vi "OldLogReader.vi"() -> ()   [LabVIEW 2011]
doc: "Processes data from status data logs. Requires the user to select the date the log was taken and the log file, then runs through it and finds each time we wrote to the log, and uses the number of times we wrote as the time. It then graphs all the information that is easily graphed and useful. Other data can be obtained by finding it in the case structure in the for loop.\n\n-By Elizabeth Mahon"
uses:
  2-Think/2 Typedefs/Velocity.ctl
  2-Think/2 Typedefs/apparent wind direction.ctl
  2-Think/2 Typedefs/apparent wind speed.ctl
  2-Think/2 Typedefs/apparent wind.ctl
  2-Think/2 Typedefs/heading.ctl
  2-Think/2 Typedefs/UTM Location.ctl
  2-Think/2 Typedefs/robot velocity.ctl
  2-Think/2 Typedefs/rate of turn.ctl
  2-Think/2 Typedefs/pitch and roll.ctl
  2-Think/2 Typedefs/generalized sensor status.ctl
  2-Think/2 Typedefs/indicator LED.ctl
  2-Think/2 Typedefs/Which Boat.ctl
  2-Think/2 Typedefs/absolute wind direction.ctl
  2-Think/2 Typedefs/absolute wind speed.ctl
  0x2-OCU-Think Comm/0x2 Typedefs/Current Waypoint.ctl
  2-Think/2 Typedefs/rudder angle.ctl
  2-Think/2 Typedefs/sail setpt.ctl
  0x2-OCU-Think Comm/0x2 Typedefs/manual override.ctl
  2-Think/2 Typedefs/setpoints to boat.ctl
  0-OCU/0 Typedefs/Maps.ctl
  <vilib>/vision/Image Controls.llb/IMAQ Image.ctl
  0-OCU/0 Typedefs/Apparent Wind Point of Sail.ctl
  0-OCU/0 Typedefs/Sail Position.ctl
  0-OCU/0 Typedefs/Rudder Position.ctl
  2-Think/2 Classes/Waypoint/Waypoint.lvclass
panel:
  in  "Overview Image Ref In":T1
  in  "Stop Replay":bool
  in  "Time":i32(slide) scale=0.0..1698.0
  out "Percent Complete":u8(slide) scale=0.0..100.0
  in  "Stop early":bool
  out "Processing File....":path
  in  "Choose graph to display":T2(tab)
  out "Sense Average":dbl
  out "Code Speed":cluster{i32[], dbl[]}[](graph)
  out "Think Average":dbl
  out "Rudder Manual?":bool
  out "Rudder Position":T3 scale=50.0..-50.0 scale format="%#.2g"
  out "Sail Manual?":bool
  in  "OCU":enum32{"Mission Map", "Detailed Telemetry"}(tab)
  out "Runprotection":bool
  out "Heading":T4 format="%05.1f"
  out "Goodness Functions Polar Plot":picture
  in  "Plot Colors":T5={"Target"=3381759, "No Sail"=16711680, "Change"=16756736, "Pure Waypt"=35080, "Pure Wind"=16860, "Combined"=16777228}
  out "Mission Map":T1(plugin-control)
  out "Apparent Wind Direction\nPoint of Sail":T6 scale=0.0..360.0 scale format="%4d"
  in  "Font Size":i16=40
  in  "Globals":T7(tab)
  out "Don't Tip?":bool
  out "Wind Sensor Status":T8
  out "Robot Heading":T4 format="%05.1f"
  out "Robot UTM Location":T10 {"North" format="%#_10f"; "East" format="%#_8f"}
  out "Robot Velocity":T11
  out "Robot\nRate of Turn":T12 format="%05.1f"
  out "Robot Pitch/Roll":T13 {"Roll" format="%05.1f"; "Pitch" format="%05.1f"}
  out "Robot Speed (m/s)":dbl
  out "Absolute Wind":T14 {"East" format="%#_5g"}
  out "Apparent Wind Direction":T15
  out "Apparent Wind Speed":T16
  out "Apparent Wind":T17
  in  "Map Name":T18="LPB Pool"
  out "Sail Position":T19
  out "Location":cluster{dbl[], dbl[]}[](graph)
  out "Battery Voltage":cluster{i32[], dbl[]}(graph)
  out "Velocity":cluster{i32[], dbl[]}[](graph)
  out "Headings":cluster{i32[], dbl[]}[](graph)
  out "Rudder":cluster{i32[], dbl[]}(graph)
  out "Sail":cluster{i32[], dbl[]}(graph)
  in  "Select date the log was taken":enum32{"Prior to 4/20/2012", "Post 4/20/2012"}(tab)
  in  "Data Log":T28 {"Current Waypoint Coords"."North" format="%#_10f"; "Current Waypoint Coords"."East" format="%#_8f"; "Robot Pitch/Roll"."Roll" format="%05.1f"; "Robot Pitch/Roll"."Pitch" format="%05.1f"; "Robot\nRate of Turn" format="%05.1f"; "Robot\nHeading" format="%05.1f"; "Robot UTM Location"."North" format="%#_10f"; "Robot UTM Location"."East" format="%#_8f"}
  in  "Data Log":T29 {"Current Waypoint Coords"."North" format="%#_10f"; "Current Waypoint Coords"."East" format="%#_8f"; "Robot Pitch/Roll"."Roll" format="%05.1f"; "Robot Pitch/Roll"."Pitch" format="%05.1f"; "Robot\nRate of Turn" format="%05.1f"; "Robot\nHeading" format="%05.1f"; "Robot UTM Location"."North" format="%#_10f"; "Robot UTM Location"."East" format="%#_8f"}
  # "NOTE: This has to be disconnected from the type def, because labview freaks out when the data taken != what this says it should be. Even in little things like type. So depending on how old the data is, you might need to change some things...."
  # "Act and network frequency are always 0.\nAs far as I can tell, network frequency is never set, so of course it's 0.\nAct, while set, is in a sequence structure where the first frame has a while loop that only ends if we e-stop, so it'll never get set."
  # "As Measured"
  # "Where Am I?"
  # "Path Planning"
  # "From Planning Functions"
  # "(this is not a cluster because subitems\nare generated in parallel code)"
  # "NOTE:\n4/20/12 - changed from Timestamp\nto string to record time"
  # "How Am I?"
  # "What's Around Me?"
  # "As Measured"
  # "As Measured"
  # "Loop Rates"
  # "Where Am I?"
  # "Path Planning"
  # "From Planning Functions"
  # "(this is not a cluster because subitems\nare generated in parallel code)"
  # "How Am I?"
  # "What's Around Me?"
  # "As Measured"
  # "As Measured"
  # "Loop Rates"
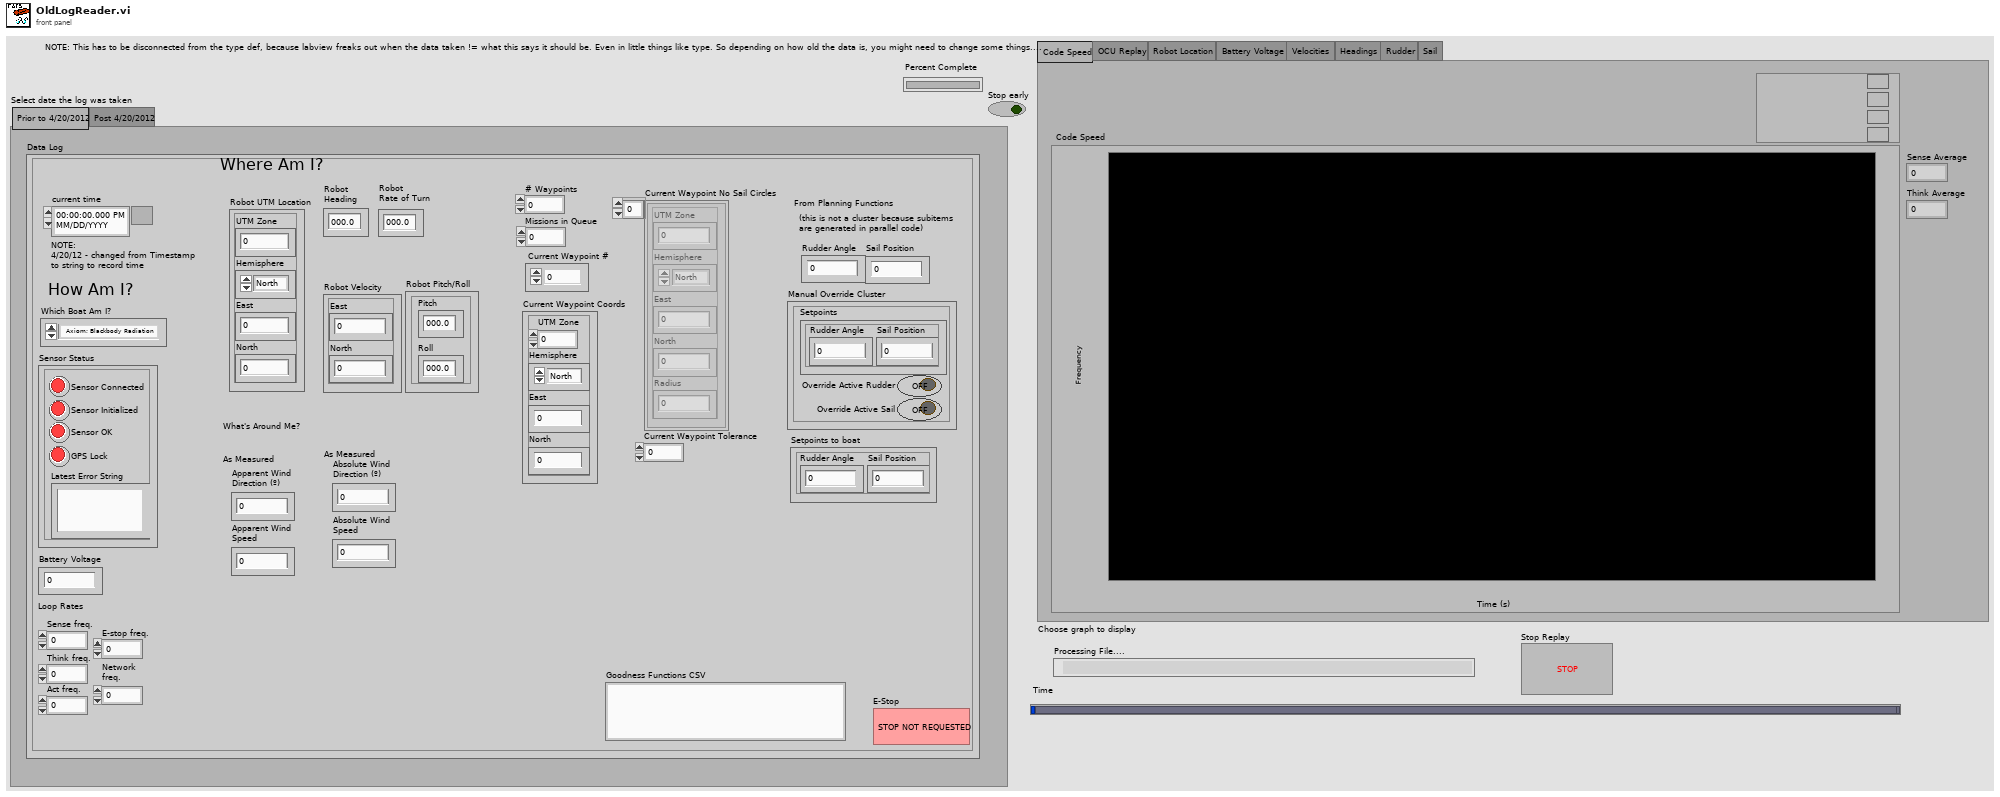
[diagram p1: front panel]
types:
  T1 = typedef "IMAQ Image.ctl" = refnum<image>
  T2 = enum32{"Code Speed", "OCU Replay", "Robot Location", "Battery Voltage", "Velocities", "Headings", "Rudder", "Sail"}
  T3 = typedef "Rudder Position.ctl" = dbl
  T4 = typedef "heading.ctl" = dbl
  T5 = cluster{"Target":u32, "No Sail":u32, "Change":u32, "Pure Waypt":u32, "Pure Wind":u32, "Combined":u32}
  T6 = typedef "Apparent Wind Point of Sail.ctl" = dbl
  T7 = enum32{"How Am I", "Where Am I", "What's Around Me"}
  T8 = typedef "generalized sensor status.ctl" = cluster{"Sensor Connected":T9, "Sensor Initialized":T9, "Sensor OK":T9, "Latest Error String":string, "GPS Lock":T9}
  T9 = typedef "indicator LED.ctl" = bool
  T10 = typedef "UTM Location.ctl" = cluster{"UTM Zone":dbl, "Hemisphere":enum16{"North", "South"}, "East":dbl, "North":dbl}
  T11 = typedef "robot velocity.ctl" = cluster{"East":dbl, "North":dbl}
  T12 = typedef "rate of turn.ctl" = dbl
  T13 = typedef "pitch and roll.ctl" = cluster{"Pitch":dbl, "Roll":dbl}
  T14 = typedef "Velocity.ctl" = cluster{"East":dbl, "North":dbl}
  T15 = typedef "apparent wind direction.ctl" = dbl
  T16 = typedef "apparent wind speed.ctl" = dbl
  T17 = typedef "apparent wind.ctl" = cluster{"Toward Fore":dbl, "Toward Starboard":dbl}
  T18 = typedef "Maps.ctl" = string
  T19 = typedef "Sail Position.ctl" = dbl
  T20 = typedef "Which Boat.ctl" = enum16{"Axiom; Blackbody Radiation", "Simulation"}
  T21 = typedef "absolute wind direction.ctl" = dbl
  T22 = typedef "absolute wind speed.ctl" = dbl
  T23 = typedef "Current Waypoint.ctl" = i32
  T24 = typedef "rudder angle.ctl" = dbl
  T25 = typedef "sail setpt.ctl" = dbl
  T26 = typedef "manual override.ctl" = cluster{"Override Active Rudder":bool, "Setpoints":T27, "Override Active Sail":bool}
  T27 = typedef "setpoints to boat.ctl" = cluster{"Sail Position":T25, "Rudder Angle":T24}
  T28 = cluster{"current time":timestamp, "Which Boat Am I?":T20, "Robot UTM Location":cluster{"UTM Zone":dbl, "Hemisphere":enum16{"North", "South"}, "East":dbl, "North":dbl}, "Robot\nHeading ":T4, "Robot\nRate of Turn":T12, "Robot Velocity":cluster{"East":dbl, "North":dbl}, "Robot Pitch/Roll":cluster{"Pitch":dbl, "Roll":dbl}, "Sensor Status":T8, "Battery Voltage":dbl, "Sense freq.":dbl, "Think freq.":dbl, "Act freq.":dbl, "E-stop freq.":dbl, "Network \nfreq.":dbl, "Apparent Wind\nDirection (º)":T15, "Apparent Wind\nSpeed":T16, "Absolute Wind\nDirection (º)":T21, "Absolute Wind\nSpeed":T22, "Missions in Queue":i32, "# Waypoints":i32, " Current Waypoint #":T23, "Current Waypoint Coords":cluster{"UTM Zone":dbl, "Hemisphere":enum16{"North", "South"}, "East":dbl, "North":dbl}, "Current Waypoint Tolerance":dbl, "Current Waypoint No Sail Circles":cluster{"UTM Zone":dbl, "Hemisphere":enum16{"North", "South"}, "East":dbl, "North":dbl, "Radius":dbl}[], "Rudder Angle":T24, "Sail Position":T25, "Manual Override Cluster":T26, "Setpoints to boat":T27, "E-Stop":bool, "Goodness Functions CSV":string}
  T29 = cluster{"Which Boat Am I?":enum16{"Competition Boat", "Small RC", "Simulation"}, "Robot UTM Location":cluster{"UTM Zone":dbl, "Hemisphere":enum16{"North", "South"}, "East":dbl, "North":dbl}, "Robot\nHeading ":T4, "Robot\nRate of Turn":T12, "Robot Velocity":cluster{"East":dbl, "North":dbl}, "Robot Pitch/Roll":cluster{"Pitch":dbl, "Roll":dbl}, "Sensor Status":T8, "Battery Voltage":dbl, "Sense freq.":dbl, "Think freq.":dbl, "Act freq.":dbl, "E-stop freq.":dbl, "Network \nfreq.":dbl, "Apparent Wind\nDirection (º)":T15, "Apparent Wind\nSpeed":T16, "Absolute Wind\nDirection (º)":T21, "Absolute Wind\nSpeed":T22, "Missions in Queue":i32, "# Waypoints":i32, " Current Waypoint #":T23, "Current Waypoint Coords":cluster{"UTM Zone":dbl, "Hemisphere":enum16{"North", "South"}, "East":dbl, "North":dbl}, "Current Waypoint Tolerance":dbl, "Current Waypoint No Sail Circles":cluster{"UTM Zone":dbl, "Hemisphere":enum16{"North", "South"}, "East":dbl, "North":dbl, "Radius":dbl}[], "Rudder Angle":T24, "Sail Position":T25, "Manual Override Cluster":T26, "Setpoints to boat":T27, "E-Stop":bool, "Goodness Functions CSV":string, "Date":string, "Time":string, "Run Protect":bool}
  T30 = cluster{"UTM Zone":dbl, "Hemisphere":enum16{"North", "South"}, "East":dbl, "North":dbl}
  T31 = cluster{"UTM Zone":dbl, "Hemisphere":enum16{"North", "South"}, "East":dbl, "North":dbl, "Radius":dbl}[]
  T32 = cluster{"UTM Zone":bool, "Hemisphere":bool, "East":bool, "North":bool}
  T33 = typedef "0-Image Descriptor.ctl" = cluster{"Upper-Left Corner Coordinates":T10, "Meters/Pixel":dbl}
  T34 = cluster{"Image Ref Out":T1, "Image Descriptor":T33}
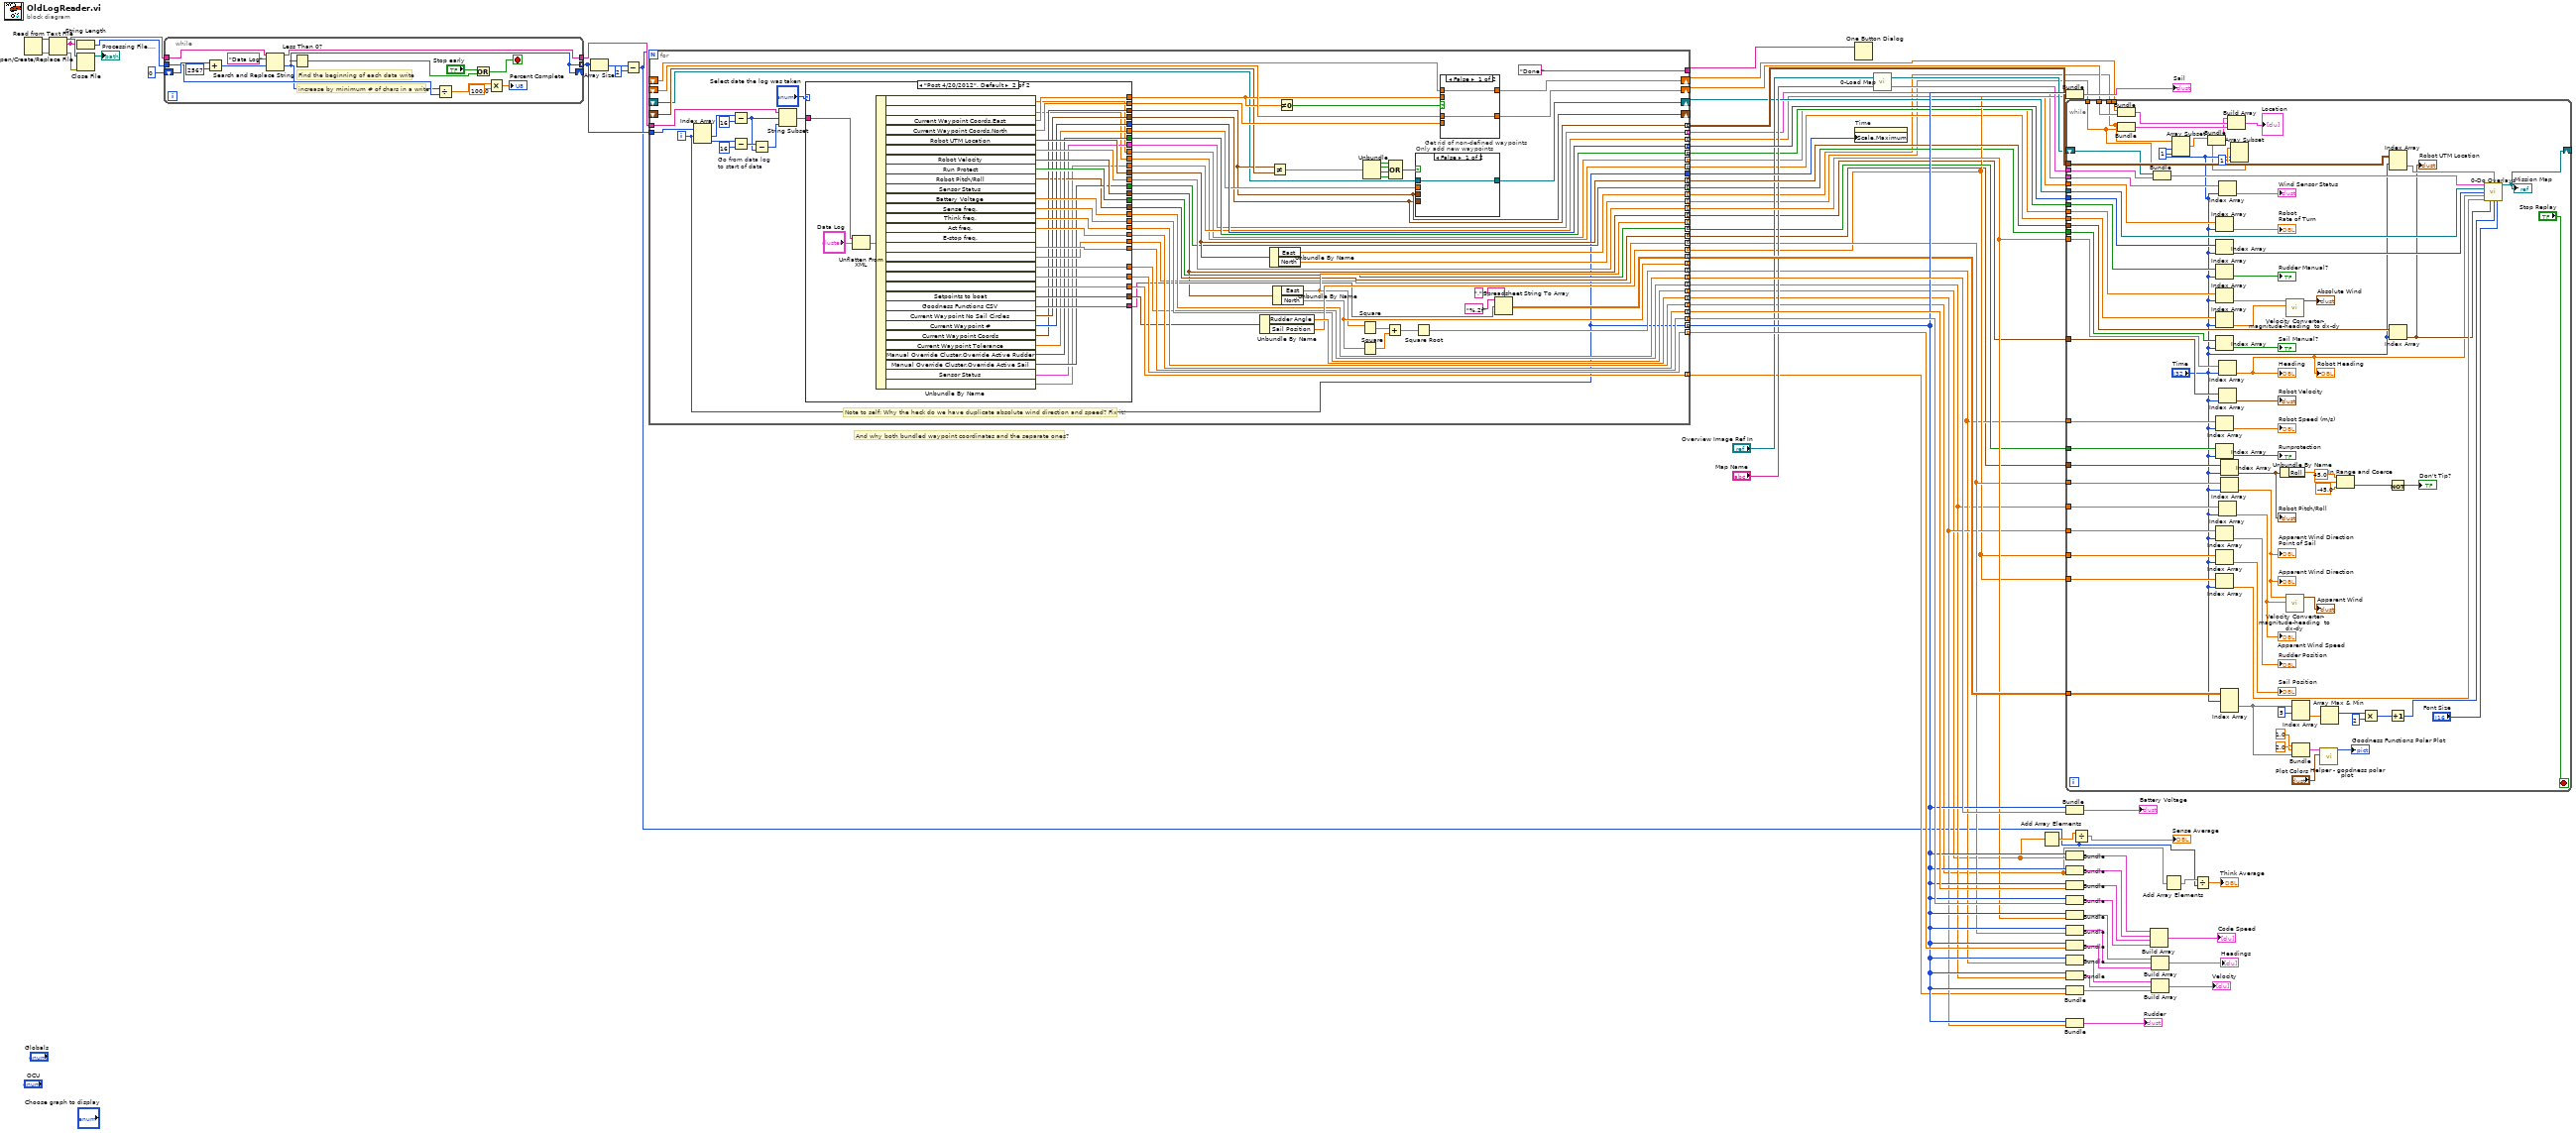
[diagram p0: block diagram]
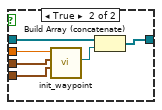
[diagram p2: hidden frame]
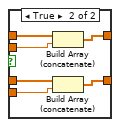
[diagram p3: hidden frame]
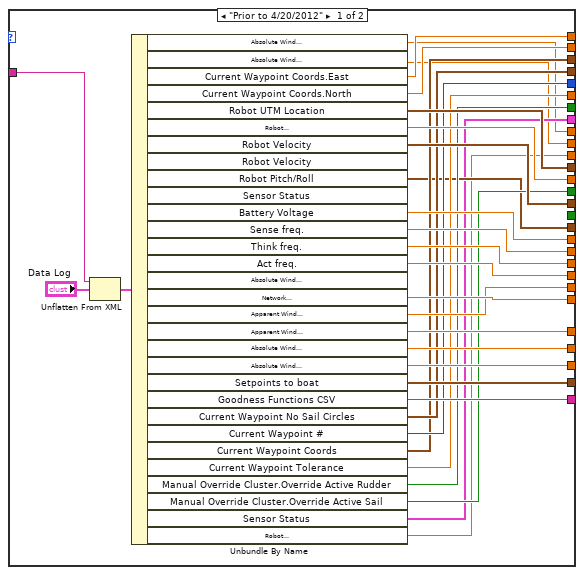
[diagram p4: hidden frame]
diagram:
  # "And why both bundled waypoint coordinates and the separate ones?"
  n1 = Open/Create/Replace File() -> (refnum out=w71:refnum<file>, error out=w42:errorcluster)  [unwired: 6 in, 1 out]
  n2 = Read from Text File(file (use dialog)=w71, error in=w42) -> (refnum out=w43:refnum<file>, text=w37:string, error out=w44:errorcluster)  [unwired: 2 in, 1 out]
  n3 = String Length(string=w37) -> (length=w36:i32)
  n4 = Close File(refnum=w43, error in=w44) -> (path=→"Processing File....":path)  [unwired: 1 out]
  n5 = while {
    tunnel: w37 -> [w75]
    shift-right: [w73] -> _
    shift-left: 0 ("offset past replacement") -> [w85]
    tunnel: [w74] -> w69
    tunnel: [w73] -> w40 mode=indexing
    tunnel: w36 -> [w77]
    stop <- w83 stop-if-true
    # "increase by minimum # of chars in a write"
    # "Find the beginning of each data write"
    n6 = Add(x=w85, y=2567) -> (x+y=w76:i32)
    n7 = Search and Replace String(input string=w75, search string="Data Log", offset=w76) -> (result string=w74:string, offset past replacement=w73:i32)  [unwired: 5 in, 2 out]
    n8 = Less Than 0?(x=w73) -> (x < 0?=w81:bool)
    n9 = Divide(x=w73, y=w77) -> (x/y=w80:dbl)
    n10 = Or(x="Stop early", y=w81) -> (x .or. y?=w83:bool)
    n11 = Multiply(x=w80, y=100.0) -> (x*y=→"Percent Complete":dbl)
  }
  n12 = Array Size(array=w40) -> (size(s)=w68:i32)
  n13 = Subtract(x=w68, y=2) -> (x-y=w2:i32)
  n14 = for {
    N: w2 -> [_]
    tunnel: w40 -> [w145]
    tunnel: w69 -> [w148]
    tunnel: [w131] -> w33 mode=indexing
    tunnel: [w130] -> w56 mode=indexing
    tunnel: [w129] -> w7 mode=indexing
    tunnel: [w128] -> w4 mode=indexing
    tunnel: [w127] -> w54 mode=indexing
    tunnel: [w126] -> w53 mode=indexing
    tunnel: [w123] -> w27 mode=indexing
    tunnel: [w125] -> w19 mode=indexing
    tunnel: [w122] -> w50 mode=indexing
    tunnel: [w124] -> w18 mode=indexing
    tunnel: [w86] -> w45 mode=indexing
    tunnel: [w141] -> w20 mode=indexing
    tunnel: [w140] -> w24 mode=indexing
    tunnel: [w139] -> w23 mode=indexing
    tunnel: [w138] -> w9 mode=indexing
    tunnel: [w137] -> w8 mode=indexing
    tunnel: ["Done!"] -> w46
    tunnel: [w135] -> _ mode=indexing
    tunnel: [w134] -> _ mode=indexing
    tunnel: [w120] -> w26 mode=indexing
    tunnel: [w116] -> w39 mode=indexing
    tunnel: [w86] -> w38
    shift-right: [w113] -> w10
    shift-left: _ -> [w112]
    shift-right: [w110] -> w11
    shift-left: _ -> [w109]
    tunnel: [w97] -> w35 mode=indexing
    tunnel: [w108] -> w34 mode=indexing
    tunnel: [w107] -> w32 mode=indexing
    shift-right: [w98] -> _
    shift-left: _ -> [w106]
    shift-right: [w96] -> w25
    shift-left: _ -> [w95]
    tunnel: [w94] -> w22 mode=indexing
    tunnel: [w93] -> w21 mode=indexing
    tunnel: [w92] -> w17 mode=indexing
    tunnel: [w91] -> w16 mode=indexing
    tunnel: [w90] -> w15 mode=indexing
    tunnel: [w89] -> w14 mode=indexing
    tunnel: [w88] -> w13 mode=indexing
    tunnel: [w87] -> w12 mode=indexing
    i -> [w86]
    # "Note to self: Why the heck do we have duplicate absolute wind direction and speed? Fix it!"
    n15 = Index Array(array=w145, index #1=w86) -> (element #1=w153:i32, element #2=w151:i32)  [unwired: 1 in]
    n16 = Subtract(x=w153, y=16) -> (x-y=w146:i32)
    n17 = Subtract "Go from data log\nto start of data"(x=w151, y=16) -> (x-y=w149:i32)
    n18 = Subtract(x=w149, y=w146) -> (x-y=w147:i32)
    n19 = String Subset(string=w148, offset (0)=w146, length (rest)=w147) -> (substring=w132:string)
    n20 = case shown="\"Post 4/20/2012\", Default" "Select date the log was taken" {
      tunnel: w132 -> [w197 w227]
      tunnel: [w196 w226] -> w107
      tunnel: [w195 w225] -> w131
      tunnel: [w194 w224] -> w90
      tunnel: [w193 w223] -> w130
      tunnel: [w192 w222] -> w129
      tunnel: [w191 w221] -> w128
      tunnel: [w190 w220] -> w127
      tunnel: [w189 w219] -> w126
      tunnel: [w188 w217] -> w125
      tunnel: [w187 w215] -> w124
      tunnel: [w186 w218] -> w123
      tunnel: [w185 w216] -> w122
      tunnel: [w183 w214] -> w121
      tunnel: [_ w213] -> w120
      tunnel: [w182 w212] -> w119
      tunnel: [w181 w211] -> w111
      tunnel: [w180 w210] -> w114
      tunnel: [w179 w209] -> w97
      tunnel: [w178 w208] -> w108
      tunnel: [w177 w207] -> w98
      tunnel: [w176 w206] -> w99
      tunnel: [w175 w205] -> w94
      tunnel: [w174 w204] -> w93
      tunnel: [w173 w203] -> w92
      tunnel: [w172 w202] -> w91
      tunnel: [w171 w201] -> w89
      tunnel: [w170 w200] -> w88
      tunnel: [w169 w199] -> w87
      frame "Prior to 4/20/2012" {
        n21 = Unflatten From XML(xml string=w197, type="Data Log") -> (value=w184:T28)  [unwired: 1 in, 1 out]
        n22 = Unbundle By Name(w184) -> ("Absolute Wind\nDirection (º)"=w170:T21, "Absolute Wind\nSpeed"=w169:T22, "Current Waypoint Coords.East"=w181:dbl, "Current Waypoint Coords.North"=w180:dbl, "Robot UTM Location"=w196:T30, "Robot\nHeading"=w195:T4, "Robot Velocity"=w194:cluster{"East":dbl, "North":dbl}, "Robot Pitch/Roll"=w173:cluster{"Pitch":dbl, "Roll":dbl}, "Battery Voltage"=w193:dbl, "Sense freq."=w192:dbl, "Think freq."=w191:dbl, "Act freq."=w190:dbl, "Network \nfreq."=w189:dbl, "Apparent Wind\nDirection (º)"=w186:T15, "Apparent Wind\nSpeed"=w188:T16, "Absolute Wind\nDirection (º)"=w185:T21, "Absolute Wind\nSpeed"=w187:T22, "Setpoints to boat"=w183:T27, "Goodness Functions CSV"=w182:string, "Current Waypoint No Sail Circles"=w179:T31, "Current Waypoint #"=w178:T23, "Current Waypoint Coords"=w177:T30, "Current Waypoint Tolerance"=w176:dbl, "Manual Override Cluster.Override Active Rudder"=w175:bool, "Manual Override Cluster.Override Active Sail"=w174:bool, "Sensor Status"=w172:T8, "Robot\nRate of Turn"=w171:T12)  [unwired: 3 out]
      }
      frame "Post 4/20/2012", Default {
        n23 = Unflatten From XML(xml string=w227, type="Data Log") -> (value=w229:T29)  [unwired: 1 in, 1 out]
        n24 = Unbundle By Name(w229) -> ("Absolute Wind\nDirection (º)"=w200:T21, "Absolute Wind\nSpeed"=w199:T22, "Current Waypoint Coords.East"=w211:dbl, "Current Waypoint Coords.North"=w210:dbl, "Robot UTM Location"=w226:T30, "Robot\nHeading"=w225:T4, "Robot Velocity"=w224:cluster{"East":dbl, "North":dbl}, "Run Protect"=w213:bool, "Robot Pitch/Roll"=w203:cluster{"Pitch":dbl, "Roll":dbl}, "Battery Voltage"=w223:dbl, "Sense freq."=w222:dbl, "Think freq."=w221:dbl, "Act freq."=w220:dbl, "Network \nfreq."=w219:dbl, "Apparent Wind\nDirection (º)"=w218:T15, "Apparent Wind\nSpeed"=w217:T16, "Absolute Wind\nDirection (º)"=w216:T21, "Absolute Wind\nSpeed"=w215:T22, "Setpoints to boat"=w214:T27, "Goodness Functions CSV"=w212:string, "Current Waypoint No Sail Circles"=w209:T31, "Current Waypoint #"=w208:T23, "Current Waypoint Coords"=w207:T30, "Current Waypoint Tolerance"=w206:dbl, "Manual Override Cluster.Override Active Rudder"=w205:bool, "Manual Override Cluster.Override Active Sail"=w204:bool, "Sensor Status"=w202:T8, "Robot\nRate of Turn"=w201:T12)  [unwired: 2 out]
      }
    }
    n25 = Unbundle By Name(w121) -> ("Rudder Angle"=w140:T24, "Sail Position"=w139:T25)
    n26 = Unbundle By Name(w107) -> ("East"=w138:dbl, "North"=w137:dbl)
    n27 = Not Equal?(x=w98, y=w106) -> (x != y?=w105:T32)
    n28 = Unbundle By Name(w90) -> ("East"=w134:dbl, "North"=w135:dbl)
    n29 = Not Equal To 0?(x=w111) -> (x != 0?=w115:bool)
    n30 = Square(x=w134) -> (x^2=w143:dbl)
    n31 = Square(x=w135) -> (x^2=w142:dbl)
    n32 = Unbundle(w105) -> ("UTM Zone"=w104:bool, "Hemisphere"=w103:bool, "East"=w102:bool, "North"=w101:bool)
    n33 = Add(x=w143, y=w142) -> (x+y=w144:dbl)
    n34 = Compound Arithmetic op=OR(w104, w103, w102, w101) -> (w100:bool)
    n35 = Square Root(x=w144) -> (sqrt(x)=w141:dbl)
    n36 = case "Only add new waypoints" shown="False" w100 {
      tunnel: w99 -> [_ w160]
      tunnel: w98 -> [_ w159]
      tunnel: w97 -> [_ w158]
      tunnel: [w154 w156] -> w96
      tunnel: w95 -> [w154 w155]
      frame False {
      }
      frame True {
        n37 = call "init_waypoint.vi"("No Sail Circles"=w158, "Coords"=w159, "Tolerance (m)"=w160) -> ("Waypoint Out"=w157:refnum<class "Waypoint.lvclass">)  [unwired: 8 in]
        n38 = Build Array (concatenate)(w155, w157) -> (w156:refnum<class "Waypoint.lvclass">[])
      }
    }
    n39 = case "Get rid of non-defined waypoints" shown="False" w115 {
      tunnel: w114 -> [_ w168]
      tunnel: [w161 w167] -> w113
      tunnel: w112 -> [w161 w166]
      tunnel: w111 -> [_ w165]
      tunnel: [w162 w164] -> w110
      tunnel: w109 -> [w162 w163]
      frame False {
      }
      frame True {
        n40 = Build Array (concatenate)(w163, w165) -> (w164:dbl[])
        n41 = Build Array (concatenate)(w166, w168) -> (w167:dbl[])
      }
    }
    n42 = Spreadsheet String To Array(delimiter (Tab)=",", format string="%.2f", spreadsheet string=w119) -> (array=w116:dbl[][])  [unwired: 1 in]
  }
  n43 = One Button Dialog(message=w46) -> ()  [unwired: 1 in, 1 out]
  n44 = property on="Time" class="Slide (strict)"("Scale.Maximum"=w38) -> ()  [unwired: 2 in, 2 out]
  n45 = call "0-Load Map.vi"("Map Name"="Map Name", "Image Ref In"="Overview Image Ref In") -> ("Image Descriptor"=w30:T33, "Image Ref Out"=w28:T1)
  n46 = Add Array Elements(numeric array=w7) -> (sum=w6:dbl)
  n47 = Bundle(w45, w23) -> (→"Sail":cluster{i32[], T25[]})  [unwired: 1 in]
  n48 = while {
    tunnel: w39 -> [w307]
    tunnel: w35 -> [w300]
    tunnel: w34 -> [w297]
    tunnel: w33 -> [w295]
    tunnel: w23 -> [w294]
    tunnel: w32 -> [w292]
    shift-right: [w284] -> _
    shift-left: w28 -> [w282]
    tunnel: w30 -> [w283]
    tunnel: w27 -> [w281]
    tunnel: w26 -> [w280]
    tunnel: w25 -> [w278]
    tunnel: w24 -> [w276]
    tunnel: w23 -> [w274]
    tunnel: w22 -> [w272]
    tunnel: w21 -> [w270]
    tunnel: w20 -> [w266]
    tunnel: w19 -> [w264]
    tunnel: w17 -> [w263]
    tunnel: w16 -> [w256]
    tunnel: w15 -> [w254]
    tunnel: w14 -> [w252]
    tunnel: w13 -> [w247]
    tunnel: w12 -> [w246]
    tunnel: w11 -> [w239]
    tunnel: w10 -> [w238]
    tunnel: w9 -> [w237]
    tunnel: w8 -> [w234]
    stop <- "Stop Replay" stop-if-true
    n49 = Bundle(w239, w238) -> (w241:cluster{dbl[], dbl[]})  [unwired: 1 in]
    n50 = Bundle(w237, w234) -> (w242:cluster{dbl[], dbl[]})  [unwired: 1 in]
    n51 = Bundle("Image Ref Out"=w282, "Image Descriptor"=w283) -> (w298:T34)  [unwired: 1 in]
    n52 = Array Subset(array=w237, index="Time", length=1) -> (w235:dbl[])
    n53 = Index Array(array=w252, index="Time") -> (element=→"Robot\nRate of Turn":T12)
    n54 = Index Array(array=w297, index="Time") -> (element=w296:T23)
    n55 = Index Array(array=w272, index="Time") -> (element=→"Rudder Manual?":bool)
    n56 = Index Array(array=w247, index="Time") -> (element=w245:T21)
    n57 = Index Array(array=w246, index="Time") -> (element=w244:T22)
    n58 = Index Array(array=w270, index="Time") -> (element=→"Sail Manual?":bool)
    n59 = Index Array(array=w266, index="Time") -> (element=→"Robot Speed (m/s)":dbl)
    n60 = Index Array(array=w280, index="Time") -> (element=→"Runprotection":bool)
    n61 = Index Array(array=w276, index="Time") -> (element=→"Rudder Position":T24)
    n62 = Index Array(array=w274, index="Time") -> (element=→"Sail Position":T25)
    n63 = Index Array(array=w294, index="Time") -> (element=w293:T25)
    n64 = Index Array(array=w256, index="Time") -> (element=→"Wind Sensor Status":T8)
    n65 = Index Array(array=w254, index="Time") -> (element=→"Robot Velocity":cluster{"East":dbl, "North":dbl})
    n66 = Index Array(array=w295, index="Time") -> (element=w267:T4)
    "Heading" <- w267
    "Robot Heading" <- w267
    n67 = Index Array(array=w264, index="Time") -> (element=w248:T16)
    "Apparent Wind Speed" <- w248
    n68 = Index Array(array=w281, index="Time") -> (element=w249:T15)
    "Apparent Wind Direction\nPoint of Sail" <- w249
    "Apparent Wind Direction" <- w249
    n69 = Index Array(array=w263, index="Time") -> (element=w262:cluster{"Pitch":dbl, "Roll":dbl})
    "Robot Pitch/Roll" <- w262
    n70 = Index Array(array=w307, index (dim 0)="Time") -> (element=w291:dbl[][])  [unwired: 2 in]
    n71 = Array Subset(array=w234, index="Time", length=1) -> (w231:dbl[])
    n72 = Bundle(w235, w231) -> (w230:cluster{dbl[], dbl[]})  [unwired: 1 in]
    n73 = Build Array(w230, w241, w242) -> (→"Location":cluster{dbl[], dbl[]}[])
    n74 = Unbundle By Name(w262) -> ("Roll"=w261:dbl)
    n75 = call "Velocity Converter- magnitude-heading  to dx-dy.vi"("Magnitude"=w244, "Heading"=w245) -> ("Vector Out"=→"Absolute Wind":T14)  [unwired: 9 in]
    n76 = call "Velocity Converter- magnitude-heading  to dx-dy.vi"("Magnitude"=w248, "Heading"=w249) -> ("Vector Out"=→"Apparent Wind":T14)  [unwired: 9 in]
    n77 = Index Array(array=w291, index (row)=5 ("disabled index (col)")) -> (element=w290:dbl[])  [unwired: 1 in]
    n78 = Bundle(1.0, 2.0, w291) -> (w303:cluster{dbl, dbl, dbl[][]})  [unwired: 1 in]
    n79 = call "Helper - goodness polar plot.vi"("Plot Colors"="Plot Colors", "Goodness Fns In"=w303) -> ("Goodness Functions Polar Plot"=→"Goodness Functions Polar Plot":picture)  [unwired: 9 in]
    n80 = Array Max & Min(array=w290) -> (max index (indices)=w289:i32)  [unwired: 3 out]
    n81 = In Range and Coerce(upper limit=45.0, x=w261, lower limit=-45.0) -> (In Range?=w258:bool)  [unwired: 1 out]
    n82 = Multiply(x=w289, y=2) -> (x*y=w287:i32)
    n83 = Not(x=w258) -> (.not. x?=→"Don't Tip?":bool)
    n84 = Increment(x=w287) -> (x+1=w286:i32)
    n85 = Index Array(array=w300, index (row)="Time") -> (element=w299:T31)  [unwired: 1 in]
    n86 = Index Array(array=w292, index="Time") -> (element=w268:T30)
    "Robot UTM Location" <- w268
    n87 = call "0-Do Overlays.vi"("Image Reference\nand Descriptor"=w298, "No Sail Circles"=w299, "Waypoints"=w278, "Current Waypoint #"=w296, "Heading"=w267, "Sail Position"=w293, "Robot UTM Location"=w268, "Optimal Heading"=w286, "Font Size"="Font Size") -> ("Image out"=w284:T1)  [unwired: 6 in]
    "Mission Map" <- w284
  }
  n88 = Bundle(w45, w56) -> (→"Battery Voltage":cluster{i32[], dbl[]})  [unwired: 1 in]
  n89 = Bundle(w45, w7) -> (w58:cluster{i32[], dbl[]})  [unwired: 1 in]
  n90 = Bundle(w45, w4) -> (w57:cluster{i32[], dbl[]})  [unwired: 1 in]
  n91 = Bundle(w45, w54) -> (w60:cluster{i32[], dbl[]})  [unwired: 1 in]
  n92 = Bundle(w45, w53) -> (w59:cluster{i32[], dbl[]})  [unwired: 1 in]
  n93 = Bundle(w45, w33) -> (w61:cluster{i32[], T4[]})  [unwired: 1 in]
  n94 = Bundle(w45, w27) -> (w62:cluster{i32[], T15[]})  [unwired: 1 in]
  n95 = Bundle(w45, w50) -> (w63:cluster{i32[], T21[]})  [unwired: 1 in]
  n96 = Bundle(w45, w20) -> (w64:cluster{i32[], dbl[]})  [unwired: 1 in]
  n97 = Bundle(w45, w19) -> (w65:cluster{i32[], T16[]})  [unwired: 1 in]
  n98 = Bundle(w45, w18) -> (w66:cluster{i32[], T22[]})  [unwired: 1 in]
  n99 = Bundle(w45, w24) -> (→"Rudder":cluster{i32[], T24[]})  [unwired: 1 in]
  n100 = Divide(x=w6, y=w2) -> (x/y=→"Sense Average":dbl)
  n101 = Build Array(w58, w57, w60, w59) -> (→"Code Speed":cluster{i32[], dbl[]}[])
  n102 = Build Array(w61, w62, w63) -> (→"Headings":cluster{i32[], T21[]}[])
  n103 = Build Array(w64, w65, w66) -> (→"Velocity":cluster{i32[], T22[]}[])
  n104 = Add Array Elements(numeric array=w4) -> (sum=w3:dbl)
  n105 = Divide(x=w3, y=w2) -> (x/y=→"Think Average":dbl)
